vi "CircleCoords.vi"(0 "Magnitude":dbl, 1 "Number of Points":i32=200, 2 "X Origin":dbl, 3 "Y Origin":dbl) -> (5 "X Coords":dbl[](array[numeric]), 6 "Y Coords":dbl[](array[numeric]))   [LabVIEW 2017]
panel:
  # "Overview: This VI Draws a circle in an XY Graph.\nRequirements: LabVIEW Full Development System.\nInstructions:\n1. Fill in the reguired Magnitude and Number of points.\n2. Use the X Origin and Y Origin to define the centre of the circle.\n2. Run the program."
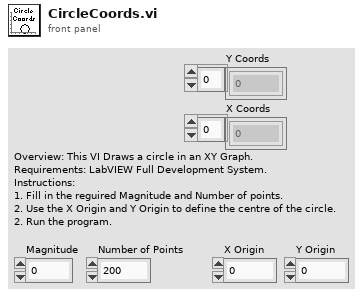
[diagram p1: front panel]
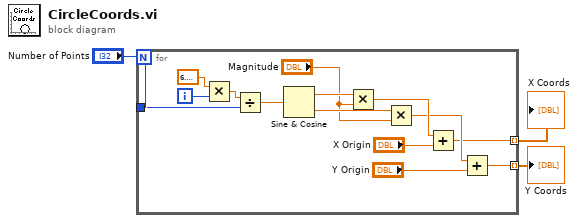
[diagram p0: block diagram]
diagram:
  n1 = for {
    N: "Number of Points" -> [_]
    tunnel: "Number of Points" -> [w15]
    tunnel: [w5] -> w1 mode=indexing
    tunnel: [w4] -> w2 mode=indexing
    i -> [w17]
    n2 = Multiply(x=6.283185307179586, y=w17) -> (x*y=w16:dbl)
    n3 = Divide(x=w16, y=w15) -> (x/y=w13:dbl)
    n4 = Sine & Cosine(0:w13) -> (1:w12:dbl, 2:w11:dbl)
    n5 = Multiply(x=w12, y="Magnitude") -> (x*y=w9:dbl)
    n6 = Multiply(x=w11, y="Magnitude") -> (x*y=w8:dbl)
    n7 = Add(x=w9, y="X Origin") -> (x+y=w5:dbl)
    n8 = Add(x=w8, y="Y Origin") -> (x+y=w4:dbl)
  }
  "Y Coords" <- w2
  "X Coords" <- w1
